vi "RSNRPZ Error-Query.vi"(8 "error in (no error)":errorcluster, 11 "VISA session":refnum<visa-resource-name> caption="VISA resource name") -> (0 "error out":errorcluster, 1 "Error Message":string, 2 "Error Code":i32, 3 "dup VISA session":refnum<visa-resource-name> caption="VISA resource name")   [LabVIEW 2010]
doc: "This VI reads an error code from the instrument's error queue."
uses:
  rsnrpz_32.dll
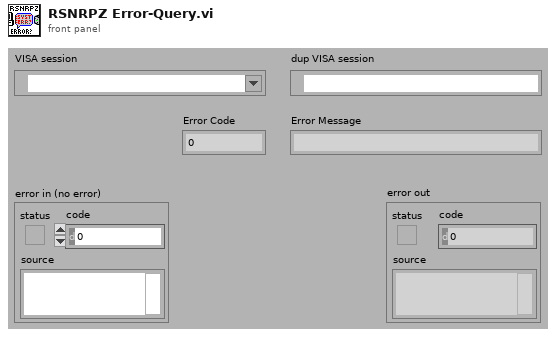
[diagram p1: front panel]
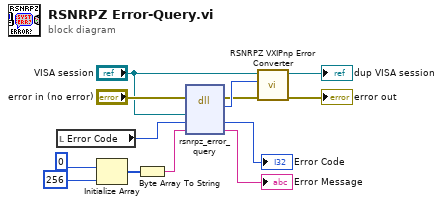
[diagram p0: block diagram]
diagram:
  n1 = local read "Error Code"() -> (w9:i32)
  n2 = Initialize Array(u8 0, 256) -> (w11:u8[])
  n3 = Byte Array To String(unsigned byte array=w11) -> (string=w7:string)
  n4 = dll-call lib="rsnrpz_32.dll" fn="rsnrpz_error_query"(error in="error in (no error)", "VISA Session"="VISA session", "Error Code"=w9, "Error Message"=w7) -> (error out=w5:errorcluster, "Status"=w10:i32, "Error Code"=→"Error Code":i32, "Error Message"=→"Error Message":string)  [unwired: 3 in, 1 out]
  n5 = call <instrlib>:"RSNRPZ VXIPnp Error Converter.vi"("error in"=w5, "VXIPnp error code"=w10, "VISA session"="VISA session") -> ("error out"=→"error out":errorcluster, "dup VISA session"=→"dup VISA session":refnum<visa-resource-name>)  [unwired: 7 in]
